vi "VCI Set Filter.vi"(7 "pFilter":T1, 9 "CANIndex":u32, 10 "DevIndex":u32, 11 "DevType":u32) -> (3 "function return":u32, 5 "pFilter out":T1)   [LabVIEW 2010, in "ControlCAN.lvlib"]
doc: "unsigned int WINAPI VCI_SetFilter(unsigned int DevType,unsigned int DevIndex,unsigned int CANIndex,PVCI_FILTER_CONFIG pFilter);"
uses:
  ControlCAN.lvlib
  ControlCAN/Ginkgo_Driver.dll
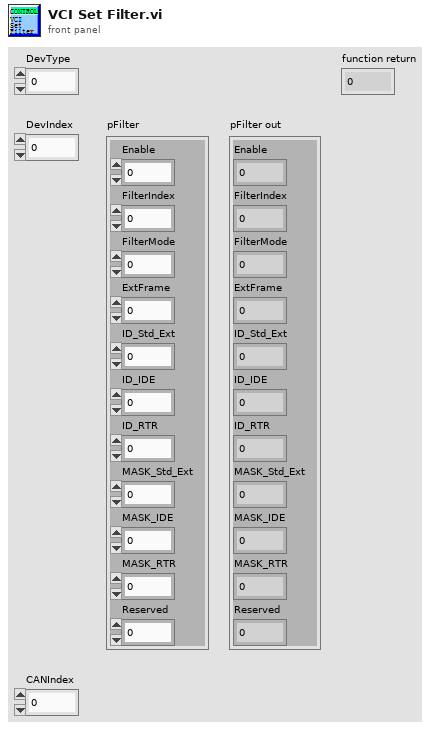
[diagram p1: front panel]
types:
  T1 = cluster{"Enable":u8, "FilterIndex":u8, "FilterMode":u8, "ExtFrame":u8, "ID_Std_Ext":u32, "ID_IDE":u32, "ID_RTR":u32, "MASK_Std_Ext":u32, "MASK_IDE":u32, "MASK_RTR":u32, "Reserved":u32}
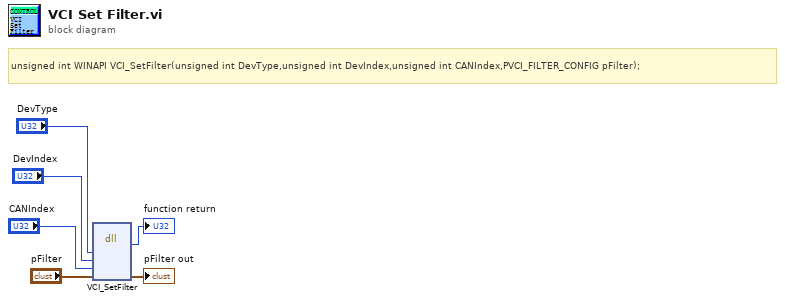
[diagram p0: block diagram]
diagram:
  # "unsigned int WINAPI VCI_SetFilter(unsigned int DevType,unsigned int DevIndex,unsigned int CANIndex,PVCI_FILTER_CONFIG pFilter);"
  n1 = dll-call lib="E:/Project/vt_ginkgo/truck/Ginkgo Driver/vs2010/Ginkgo_USB-I2C&SPI&CAN_API_v2.0.3.3/lib/labview_32bit/ControlCAN/Ginkgo_Driver.*" fn="VCI_SetFilter"("DevType"="DevType", "DevIndex"="DevIndex", "CANIndex"="CANIndex", "pFilter"="pFilter") -> (→"function return":u32, "pFilter"=→"pFilter out":T1)  [unwired: 6 in, 2 out]
